vi "PXI_Host_LargeFXP_Read_OldMethod_Benchmark.vi"() -> ()   [LabVIEW 2018]
uses:
  <vilib>/Platform/TimedLoop/XDataNode/timing_clust.ctl
  <vilib>/Platform/TimedLoop/XDataNode/nitl_modes.ctl
  <vilib>/Platform/TimedLoop/XDataNode/wakeup.ctl
  <vilib>/addons/FPGA Advanced Session Resources/LVFPGA Adv Session Resources/OpenByNameSubVI.vi
  <vilib>/rvi/interface/common/dynamic/niFpgaEscapeDelimiterAndNull.vi
  <vilib>/Utility/error.llb/Error Cluster From Error Code.vi
  <vilib>/rvi/errors/niLvFpgaAdjustHostInterfaceError.vi
  <vilib>/FPGAPlugInAG/Dynamic/niLvFpga_Close_Dynamic.vi
  <vilib>/addons/FPGA Advanced Session Resources/LVFPGA Adv Session Resources/OpenByName.xnode
  <vilib>/platform/TimedLoop/XDataNode/XDataNode.xnode
  <vilib>/rvi/interface/nirviReadWriteControl/nirviReadWriteControl.xnode
  <vilib>/rvi/interface/nirviCloseFPGA/nirviCloseFPGA.xnode
  NiFpgaLv.dll
  <vilib>/rvi/interface/Simulation/niFpgaSimulationCallBeginRW.vi
  <vilib>/addons/FPGA Advanced Session Resources/LVFPGA Adv Session Resources/LVFPGAAdvSessionResources.lvlib
  <vilib>/Platform/TimedLoop/XDataNode/XDNodeRunTimeDep.lvlib
panel:
  out "Waveform Graph":dbl[](graph)
  out "Standard Dev":dbl
  out "Arithmetic Mean":dbl
  out "Maximum":dbl
  out "Value out":fxp<+/-,64,12>
  out "error out":errorcluster
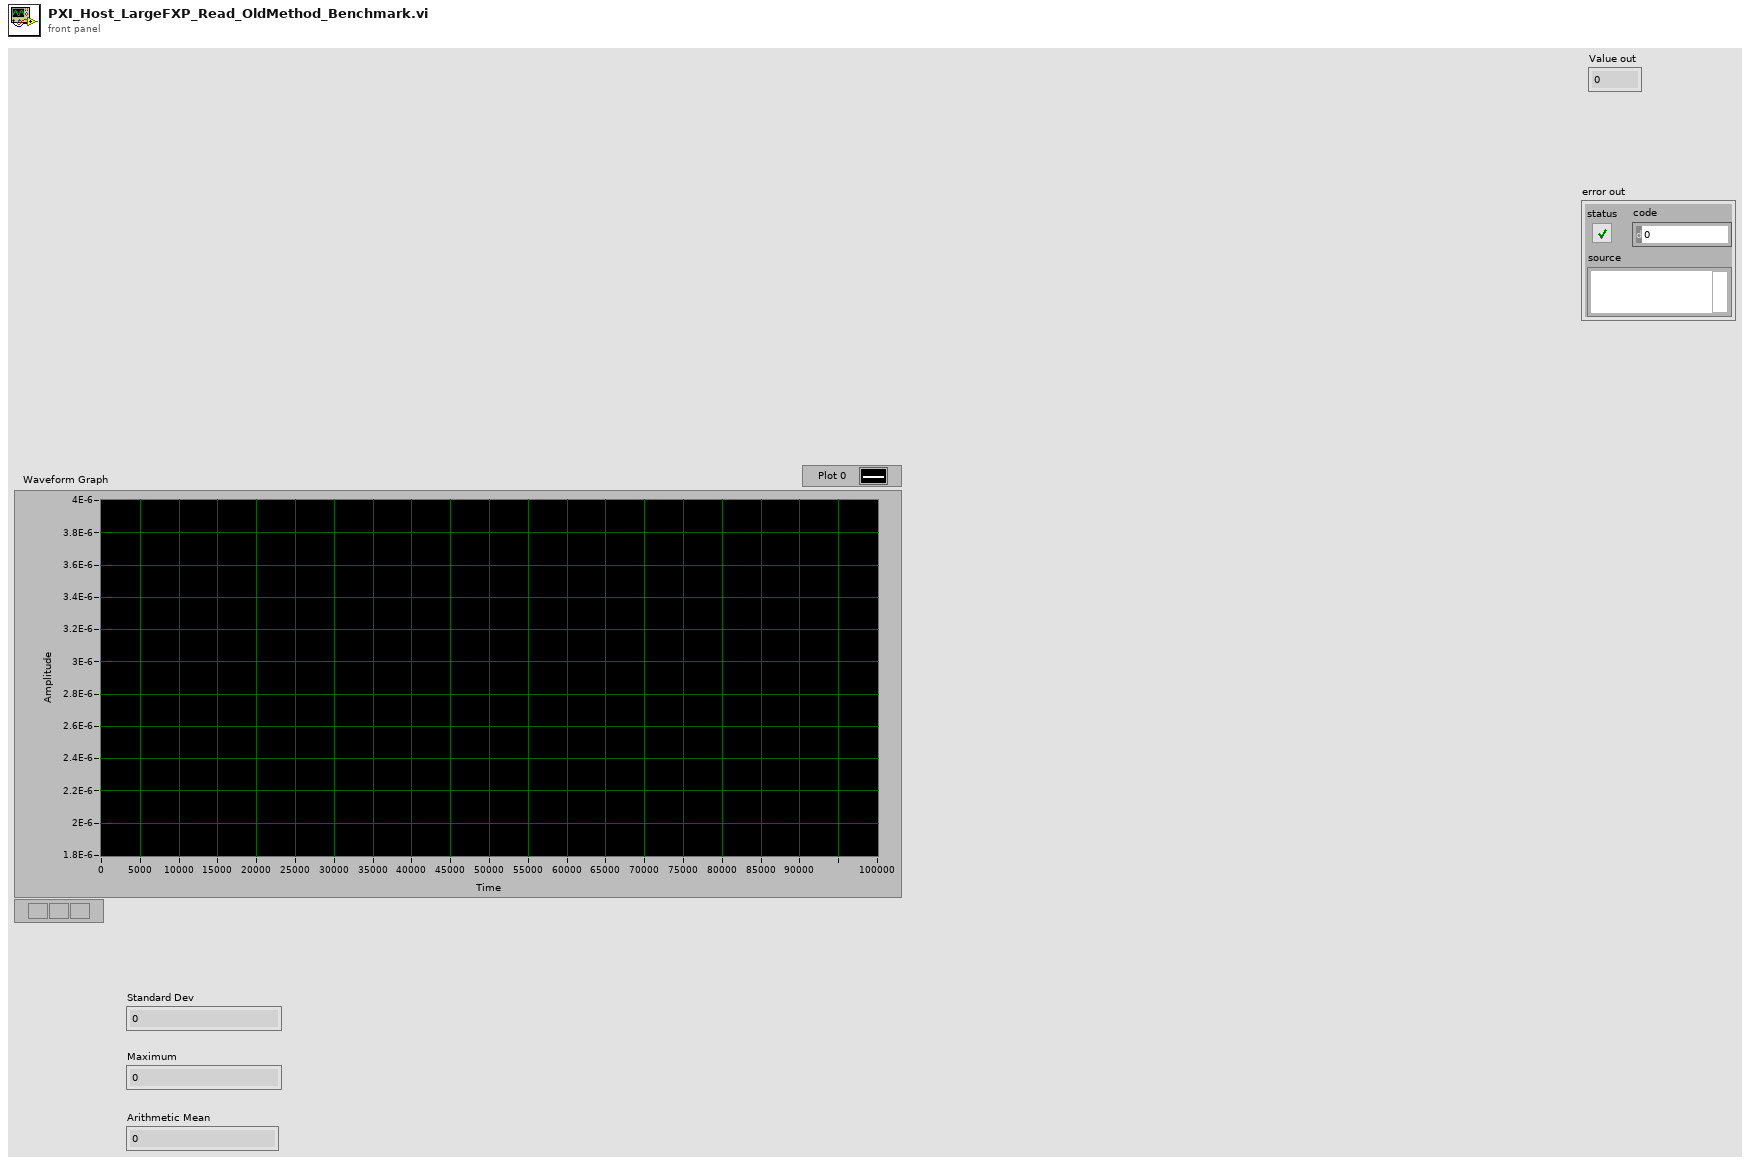
[diagram p1: front panel]
types:
  T1 = typedef "XDNodeRunTimeDep.lvlib/timing_clust.ctl" = cluster{"Expected End [f-1]":u64, "Actual End [f-1]":u64, "Finished Late? [f-1]":bool, "Expected End [i-1]":u64, "Actual End [i-1]":u64, "Finished Late? [i-1]":bool, "Expected Start [i]":u64, "Actual Start [i]":u64, "Expected Start [f]":u64, "Actual Start [f]":u64, "Source Name":string, "Structure Name":string, "Period":i64, "Deadline":i64, "Offset":i64, "Start":i64, "Priority":i32, "Timeout":i32, "Mode":T2, "Wakeup Reason":T3, "Error":errorcluster, "Source Type":string, "Secondary Source Type":string, "Global End Time":u64, "Global Start Time":u64, "Frame Duration":u64, "Iteration Duration":u64, "Assigned CPU":i32, "I/O Scan Engine Mode":u32}
  T2 = typedef "XDNodeRunTimeDep.lvlib/nitl_modes.ctl" = enum32{"No Change", "Process missed periods, maintain original phase", "Discard missed periods, maintain original phase", "Process missed periods, ignore original phase", "Discard missed periods, ignore original phase"}
  T3 = typedef "XDNodeRunTimeDep.lvlib/wakeup.ctl" = enum32{"Normal", "Aborted", "Asynchronous wakeup", "Timing source error", "Timed loop error", "Timeout"}
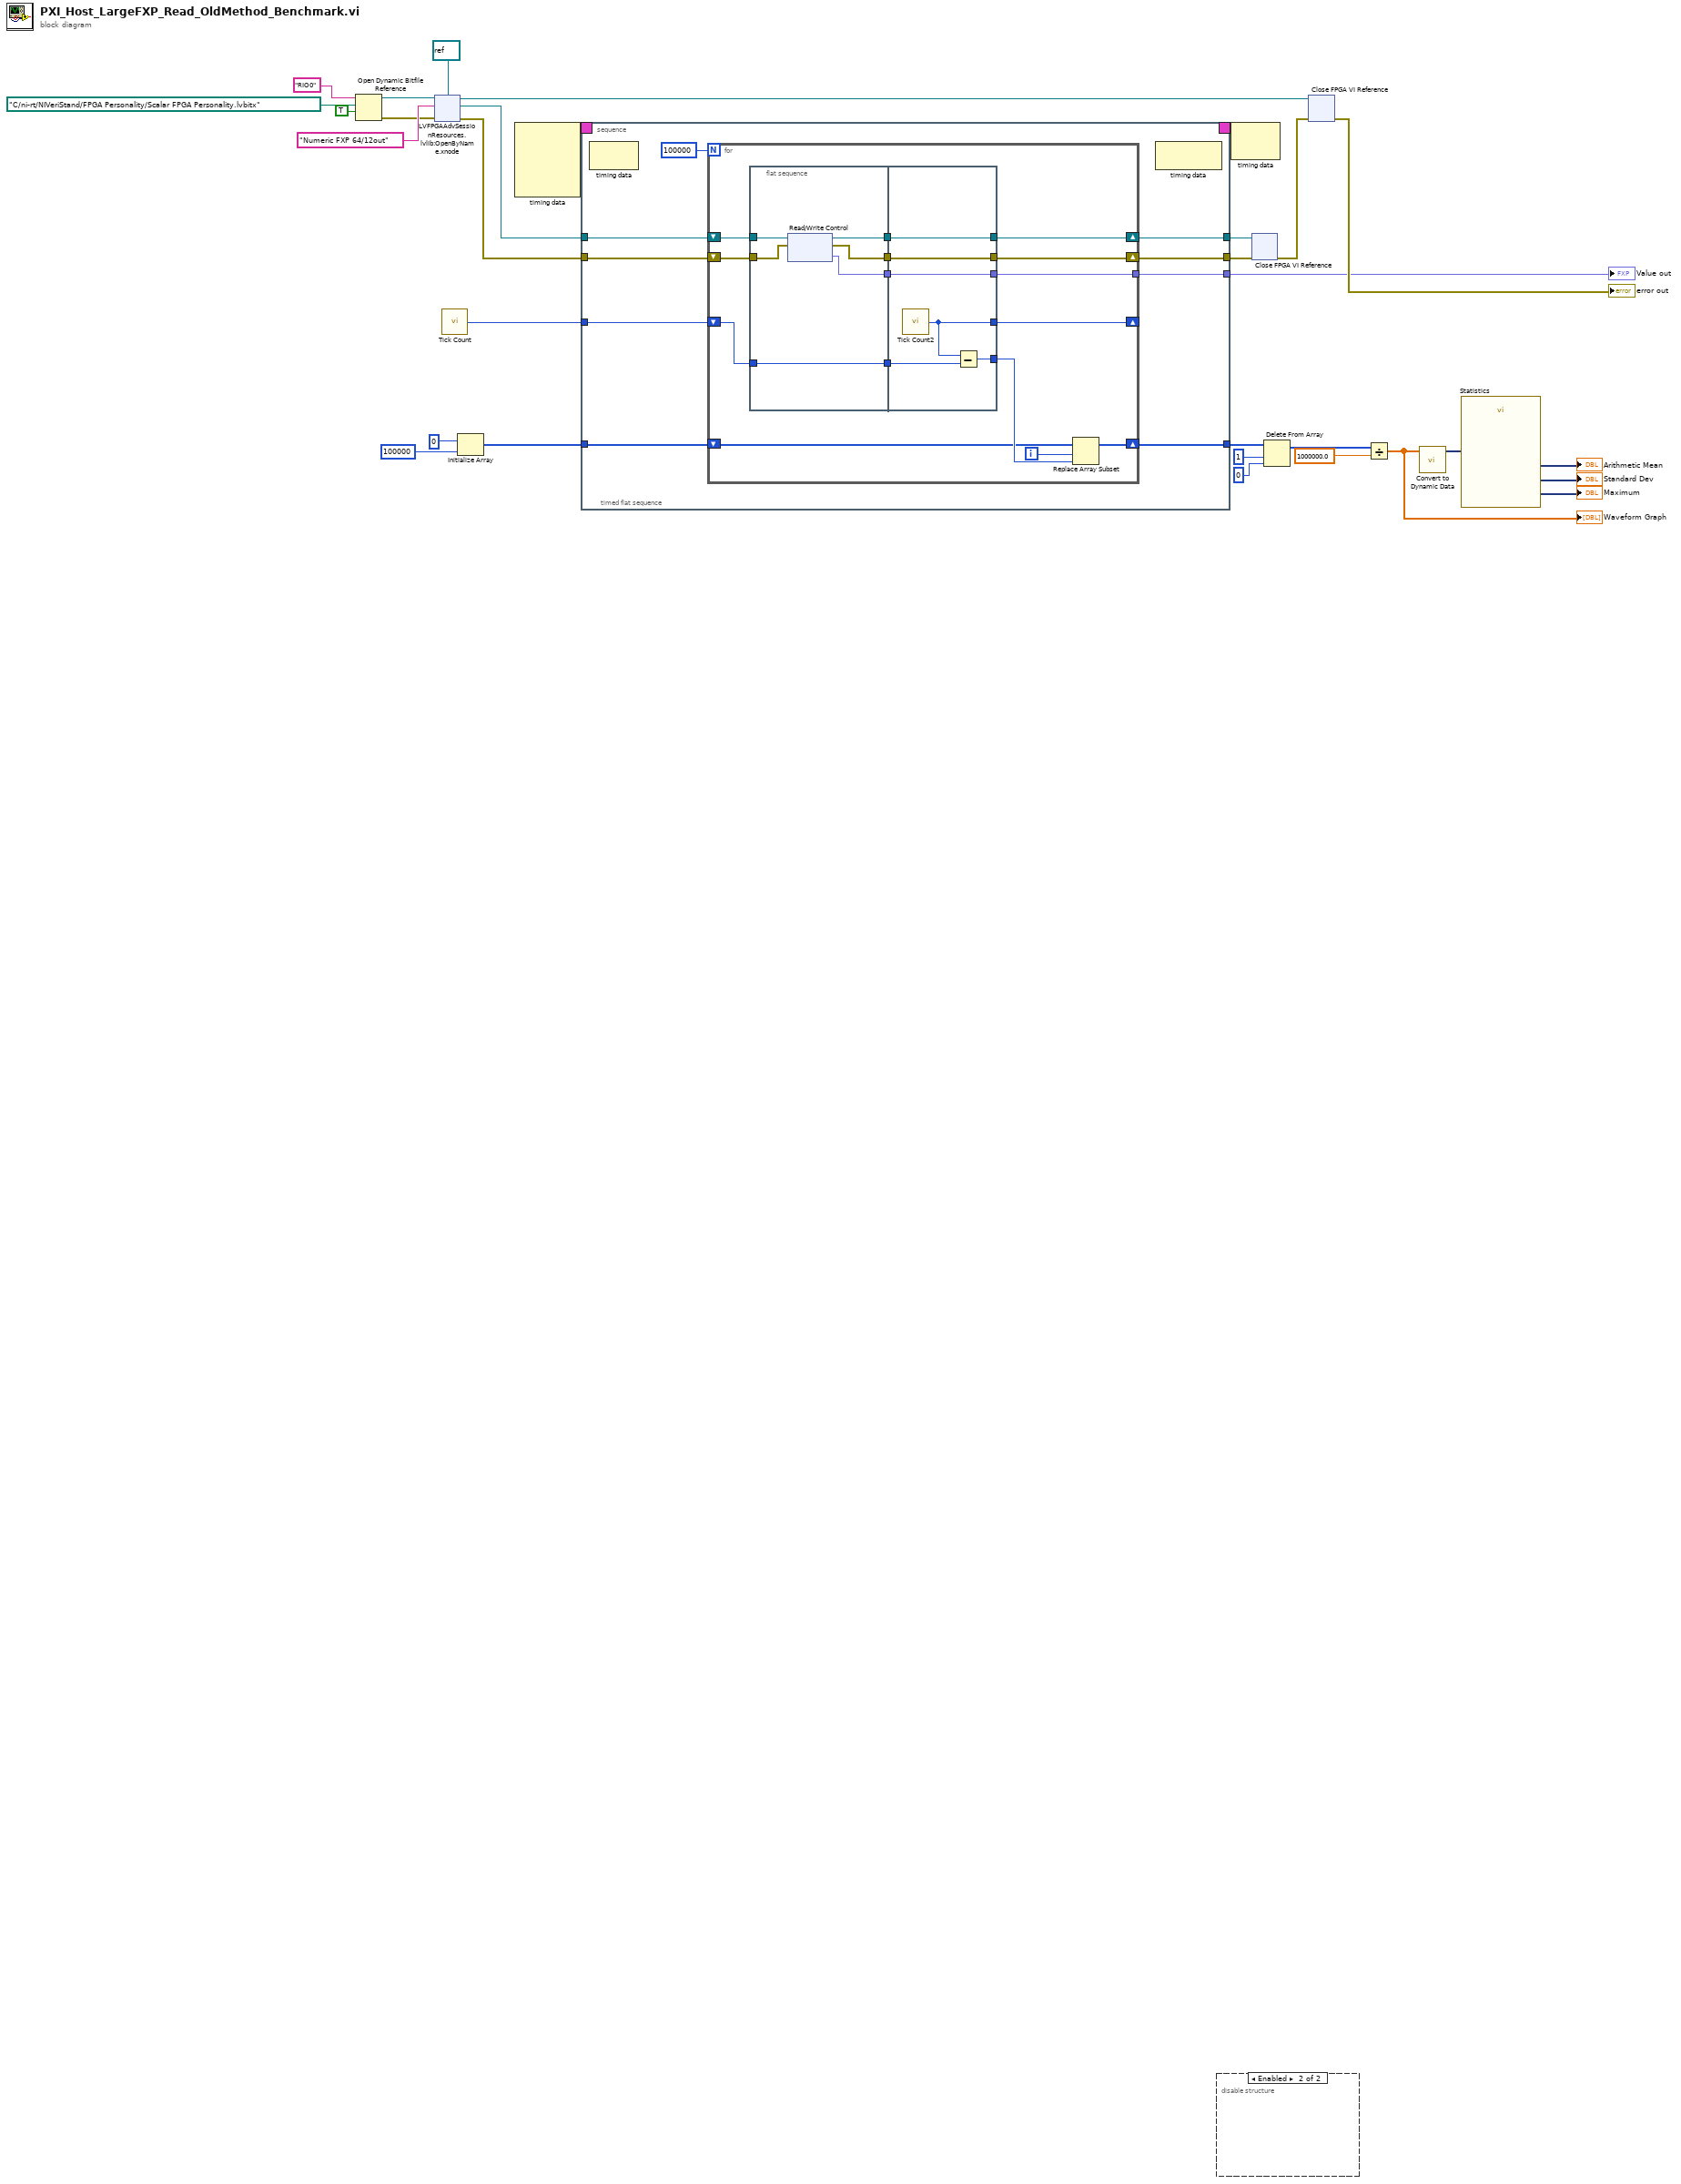
[diagram p0: block diagram]
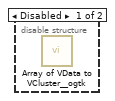
[diagram p2: hidden frame]
diagram:
  n1 = Open Dynamic Bitfile Reference(0:"RIO0" ("Device address"), 1:path "C:/ni-rt/NIVeriStand/FPGA Personality/Scalar FPGA Personality.lvbitx" ("Bitfile path"), 2:TRUE ("Run When Loaded")) -> (5:w27:refnum<k20>, 8:w25:errorcluster)  [unwired: 2 in]
  n2 = xnode "LVFPGAAdvSessionResources.lvlib:OpenByName.xnode"("FPGA VI Reference in"=w27, "Resource name in"="Numeric FXP 64/12out", "Single resource reference type in"=refnum<k20> refnum ("Type"), "Error in"=w25) -> ("Single resource reference out"=w23:refnum<k20>, "Error out"=w24:errorcluster, "FPGA VI Reference out"=w19:refnum<k20>)
  n3 = call "Tick Count"() -> ("Tick Count(uSec)"=w14:u32)
  n4 = Initialize Array(u32 0 ("Tick Count(uSec)"), 100000) -> (w2:u32[])
  n5 = node-c288() -> (w16:T1)  [unwired: 4 in]
  n6 = timed-sequence {
    timing: w16 -> [_]
    timing-out: [_] -> w15
    tunnel: [w39] -> w28
    tunnel: w24 -> [w38]
    tunnel: w23 -> [w37]
    tunnel: [w36] -> w21
    tunnel: [w35] -> w17
    tunnel: w14 -> [w34]
    tunnel: w2 -> [w33]
    tunnel: [w32] -> w1
    n7 = timed-flat-sequence {
      tunnel: [w48] -> w39
      tunnel: w38 -> [w47]
      tunnel: w37 -> [w46]
      tunnel: [w45] -> w36
      tunnel: [w44] -> w35
      tunnel: w34 -> [w42]
      tunnel: w33 -> [w41]
      tunnel: [w40] -> w32
      n8 = node-c288() -> ()  [unwired: 1 in, 1 out]
      n9 = for {
        N: 100000 -> [_]
        tunnel: [w58] -> w44
        shift-right: [w62] -> w48
        shift-left: w47 -> [w61]
        shift-right: [w59] -> w45
        shift-left: w46 -> [w60]
        shift-right: [w55] -> _
        shift-left: w42 -> [w57]
        shift-right: [w51] -> w40
        shift-left: w41 -> [w52]
        i -> [w53]
        n10 = flat-sequence {
          tunnel: [w69] -> w65
          tunnel: [w68] -> w64
          tunnel: [w67] -> w63
          tunnel: w60 -> [w71]
          tunnel: w61 -> [w70]
          tunnel: w57 -> [w66]
          tunnel: [w66] -> w56
          tunnel: [w77] -> w54
          tunnel: w65 -> [w76]
          tunnel: [w76] -> w62
          tunnel: [w75] -> w58
          tunnel: w64 -> [w75]
          tunnel: w63 -> [w74]
          tunnel: [w74] -> w59
          tunnel: w56 -> [w73]
          tunnel: [w72] -> w55
          frame #0 {
            n11 = xnode "Read/Write Control"("FPGA VI Reference In"=w71, "error in"=w70) -> ("FPGA VI Reference Out"=w67:refnum<k20>, "error out"=w69:errorcluster, "Value"=w68:fxp<+/-,64,12>)
          }
          frame #1 {
            n12 = call "Tick Count2"() -> ("Tick Count(uSec)"=w72:u32)
            n13 = Subtract(x=w72, y=w73) -> (x-y=w77:u32)
          }
        }
        n14 = Replace Array Subset(array=w52, new element=w54, index=w53) -> (w51:u32[])
      }
      n15 = node-c288() -> ()  [unwired: 1 in, 1 out]
    }
  }
  "Value out" <- w17
  n16 = disable-structure shown="Enabled" {
    frame Disabled {
      n17 = call <userlib>:"Array of VData to VCluster__ogtk.vi"() -> ()  [unwired: 10 in, 2 out]
    }
    frame Enabled {
    }
  }
  n18 = node-c288(w15) -> ()  [unwired: 1 out]
  n19 = xnode "Close FPGA VI Reference"("FPGA VI Reference In"=w21, "error in"=w28) -> ("error out"=w20:errorcluster)
  n20 = Delete From Array(array=w1, length=1, index=0) -> (array with subset deleted=w3:u32[])  [unwired: 1 out]
  n21 = xnode "Close FPGA VI Reference"("FPGA VI Reference In"=w19, "error in"=w20) -> ("error out"=→"error out":errorcluster)
  n22 = Divide(x=w3, y=1000000.0) -> (x/y=w4:dbl[])
  "Waveform Graph" <- w4
  n23 = call "Convert to Dynamic Data"("Array"=w4) -> ("Dynamic Data Type"=w11:dynamicdata)  [unwired: 3 in]
  n24 = call "Statistics"("Signals"=w11) -> ("Standard Dev"=→"Standard Dev":dynamicdata, "Arithmetic Mean"=→"Arithmetic Mean":dynamicdata, "Maximum"=→"Maximum":dynamicdata)  [unwired: 23 in, 1 out]
